vi "Write Analog Out State.vi"(8 "error in":errorcluster, 9 "Selection":i32, 10 "Value":dbl, 11 "PLC in":refnum<class "PLC.lvclass">) -> (0 "error out":errorcluster, 3 "PLC out":refnum<class "PLC.lvclass">)   [LabVIEW 2018, in "PLC.lvlib" / "PLC.lvclass"]
uses:
  PLC.lvclass
  Custom Controls/Selector.ctl
  PLC.lvclass/PLC.ctl
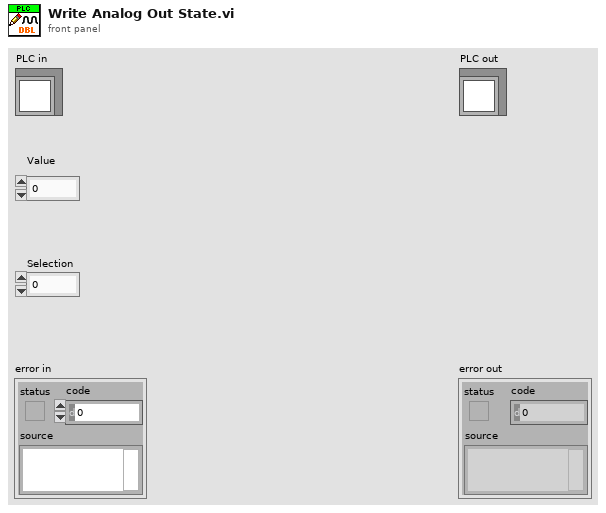
[diagram p1: front panel]
types:
  T1 = typedef "PLC.lvlib/PLC.lvclass/Selector.ctl" = enum16{"Digital", "Analog"}
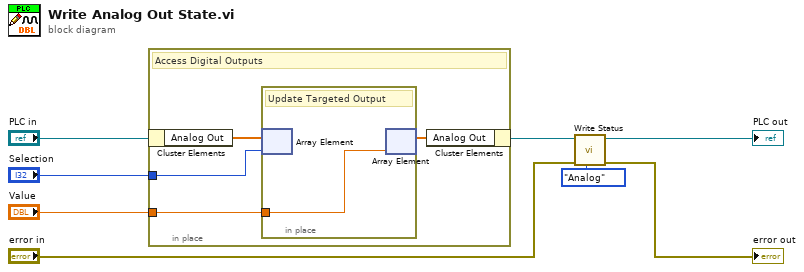
[diagram p0: block diagram]
diagram:
  n1 = in-place {
    in-place-border: "Selection" -> [w10]
    in-place-border: "Value" -> [w9]
    # "Access Digital Outputs"
    n2 = in-place-cluster #1("PLC in") -> ("Analog Out"=w12:dbl[])
    n3 = in-place {
      in-place-border: w9 -> [w13]
      # "Update Targeted Output"
      n4 = in-place-array #2(w12, w10) -> ()  [unwired: 1 out]
      n5 = in-place-array #2(w13) -> (w11:dbl[])  [unwired: 1 out]
    }
    n6 = in-place-cluster #1("Analog Out"=w11) -> (w7:refnum<class "PLC.lvclass">)
  }
  n7 = call-dynamic "Write Status.vi"("Selector"=Selector."Analog", "error in"="error in", "PLC in"=w7) -> ("error out"=→"error out":errorcluster, "PLC out"=→"PLC out":refnum<class "PLC.lvclass">)  [unwired: 7 in]
